vi "DO Update.vi"(8 "error in":errorcluster, 10 "Interupt Q":refnum<queue>, 11 "DO Config Data":T1) -> (0 "error out":errorcluster, 1 "Data to Generate":bool[](array[boolean]), 2 "Stop":bool, 3 "DO Config Data 2":T1)   [LabVIEW 2024]
doc: "All Rights Reserved © 2017 SyncSols"
uses:
  TCP Engine/Controls/TCP Engine I&O  Interupt Cluster.ctl
  Host-DQMH/Configuration/DO Channel's.ctl
  Controls/DO Update Cluster.ctl
  TCP Engine/TCP Engine.lvlib
  Host-DQMH/Configuration/Configuration.lvlib
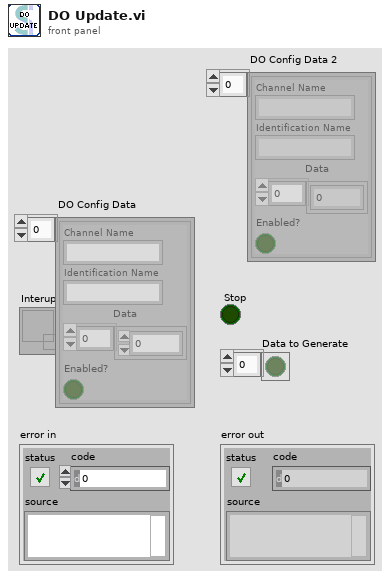
[diagram p1: front panel]
types:
  T1 = typedef "Configuration.lvlib/DO Channel's.ctl" = cluster{"Channel Name":string, "Identification Name":string, "Data":u8[], "Enabled?":bool}[]
  T2 = typedef "DO Update Cluster.ctl" = cluster{"Channel":string[], "Data":u8[]}
  T3 = typedef "TCP Engine.lvlib/TCP Engine I&O  Interupt Cluster.ctl" = cluster{" Stop":bool, "JSON Variant":variant}
  T4 = cluster{"Channel Name":string, "Identification Name":string, "Data":u8[], "Enabled?":bool}
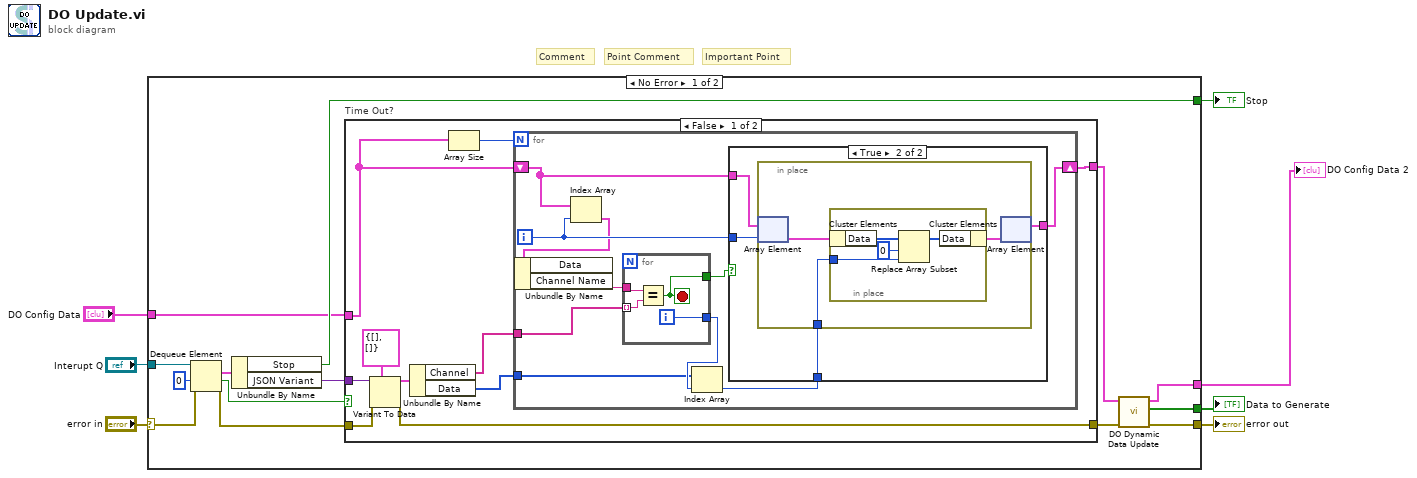
[diagram p0: block diagram]
diagram:
  # "Important Point"
  # "Point Comment"
  # "Comment"
  n1 = case shown="No Error" "error in" {
    selector: "error in" -> [w18 w61]
    tunnel: [w12 w61] -> w7
    tunnel: "Interupt Q" -> [w19 _]
    tunnel: [w14 _] -> w4
    tunnel: [w10 w60] -> w2
    tunnel: [w9 _] -> w3
    tunnel: "DO Config Data" -> [w8 w60]
    frame No Error {
      n2 = Dequeue Element(queue=w19, timeout in ms (-1)=0, error in (no error)=w18) -> (element=w20:T3, timed out?=w17:bool, error out=w16:errorcluster)  [unwired: 1 out]
      n3 = Unbundle By Name(w20) -> ("Stop"=w14:bool, "JSON Variant"=w15:variant)
      n4 = case "Time Out?" shown="False" w17 {
        tunnel: w16 -> [w31 w59]
        tunnel: w15 -> [w30 _]
        tunnel: w8 -> [w24 w58]
        tunnel: [w26 w59] -> w13
        tunnel: [w25 w58] -> w11
        frame False {
          n5 = Variant To Data(error in=w31, type=T2 {"Channel"=[], "Data"=[]} ("DO Update Cluster"), Variant=w30) -> (data=w28:T2, error out=w26:errorcluster)
          n6 = Unbundle By Name(w28) -> ("Channel"=w27:string[], "Data"=w22:u8[])
          n7 = Array Size(array=w24) -> (size(s)=w23:i32)
          n8 = for {
            N: w23 -> [_]
            tunnel: w27 -> [w40]
            shift-right: [w38] -> w25
            shift-left: w24 -> [w37]
            tunnel: w22 -> [w33]
            i -> [w36]
            n9 = Index Array(array=w37, index=w36) -> (element=w35:T4)
            n10 = Unbundle By Name(w35) -> ("Channel Name"=w41:string)  [unwired: 1 out]
            n11 = for {
              tunnel: w41 -> [w57]
              tunnel: w40 -> [w56] mode=indexing
              tunnel: [w55] -> w39
              tunnel: [w54] -> w34
              i -> [w54]
              stop <- w55 stop-if-true
              n12 = Equal?(x=w57, y=w56) -> (x = y?=w55:bool)
            }
            n13 = Index Array(array=w33, index=w34) -> (element=w32:u8)
            n14 = case shown="True" w39 {
              tunnel: w36 -> [_ w44]
              tunnel: w32 -> [_ w46]
              tunnel: w37 -> [w42 w45]
              tunnel: [w42 w43] -> w38
              frame False {
              }
              frame True {
                n15 = in-place {
                  in-place-border: w46 -> [w49]
                  n16 = in-place-array #1(w45, w44) -> (w48:T4)
                  n17 = in-place {
                    in-place-border: w49 -> [w52]
                    n18 = in-place-cluster #2(w48) -> ("Data"=w53:u8[])
                    n19 = Replace Array Subset(array=w53, new element=w52, index=0) -> (w50:u8[])
                    n20 = in-place-cluster #2("Data"=w50) -> (w47:T4)
                  }
                  n21 = in-place-array #1(w47) -> (w43:T1)  [unwired: 1 out]
                }
              }
            }
          }
        }
        frame True {
        }
      }
      n22 = call "DO Dynamic Data Update.vi"("error in"=w13, "DO Config Data"=w11) -> ("error out"=w12:errorcluster, "Data to Generate"=w9:bool[], "DO Config Data 2"=w10:T1)  [unwired: 7 in]
    }
    frame Error {
    }
  }
  "error out" <- w7
  "Stop" <- w4
  "Data to Generate" <- w3
  "DO Config Data 2" <- w2
